vi "PCA9525 - CJB.vi"(8 "error in (no error)":errorcluster, 10 "buffer":u8[](array[numeric])=[2, 255, 255], 11 "handle":u64 format="%x") -> (0 "error out":errorcluster, 3 "handle out":u64)   [LabVIEW 2024]
doc: "Control of CJB on RIB Tickler\nAll relay are set to an output then a buffer can be edited to control which relays are high and low."
panel:
  out "sizeTransferred (Output) 2":u32
  out "sizeTransferred (Output)":u32
  # "CJB Control"
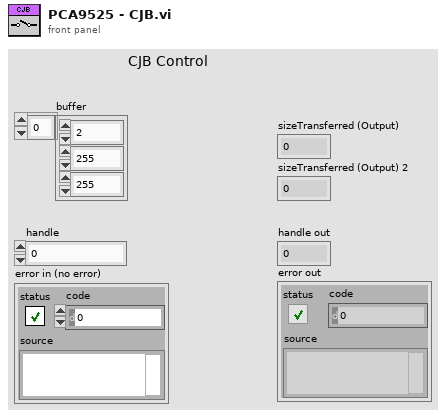
[diagram p1: front panel]
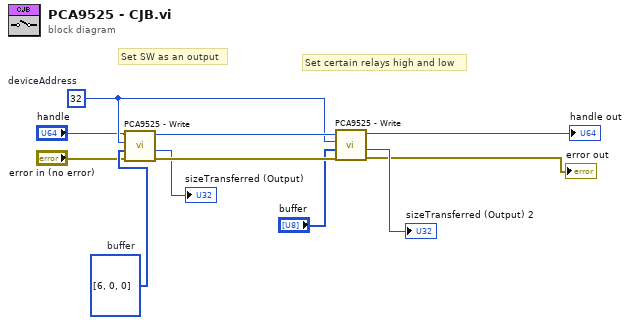
[diagram p0: block diagram]
diagram:
  w9 = u8 32  # deviceAddress
  w7 = u8[] [6, 0, 0]  # buffer
  # "Set certain relays high and low"
  # "Set SW as an output"
  n1 = call "PCA9525 - Write.vi"("error in (no error)"="error in (no error)", "buffer"=w7, "deviceAddress"=w9, "handle"="handle") -> ("error out"=w10:errorcluster, "sizeTransferred (Output)"=→"sizeTransferred (Output)":u32, "handle 2"=w11:u64)  [unwired: 4 in, 1 out]
  n2 = call "PCA9525 - Write.vi"("error in (no error)"=w10, "buffer"="buffer", "deviceAddress"=w9, "handle"=w11) -> ("error out"=→"error out":errorcluster, "sizeTransferred (Output)"=→"sizeTransferred (Output) 2":u32, "handle 2"=→"handle out":u64)  [unwired: 4 in, 1 out]
